vi "send Predef Init LV.vi"(9 "freq":u16, 10 "selection":u16, 11 "instance":i32) -> ()   [LabVIEW 2023, in "SADI_FW3.lvlib"]
doc: "SADI_API_Wrapper void sendPredefInit_LV(int instance,uint16_t selection, uint16_t freq);"
uses:
  SADI_FW3.lvlib
  SADI_FW3.dll
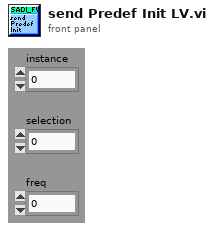
[diagram p1: front panel]
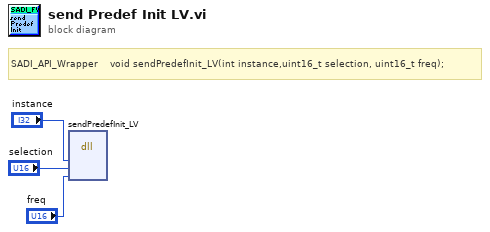
[diagram p0: block diagram]
diagram:
  # "SADI_API_Wrapper    void sendPredefInit_LV(int instance,uint16_t selection, uint16_t freq);"
  n1 = dll-call lib="C:/Users/loran/Documents/School/24_Spring/Controls Lab/EML4314c_Sp24_framework_0/LVLib/SADI_FW3.*" fn="sendPredefInit_LV"("instance"="instance", "selection"="selection", "freq"="freq") -> ()  [unwired: 7 in, 2 out]
